vi "Test Create (From VI Reference).vi"(8 "error in (no error)":errorcluster) -> (0 "error out":errorcluster)   [LabVIEW 2020, in "TEST JKI State Machine API.lvlib"]
uses:
  TEST JKI State Machine API.lvlib
  <vilib>/addons/_JKI Toolkits/Caraya/classes/Assert/Assert.lvclass
  <vilib>/addons/_JKI Toolkits/Caraya/classes/Test/Test.lvclass
  source/JKI SM/JKI SM.lvclass
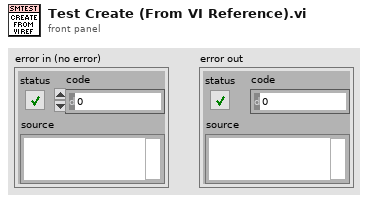
[diagram p1: front panel]
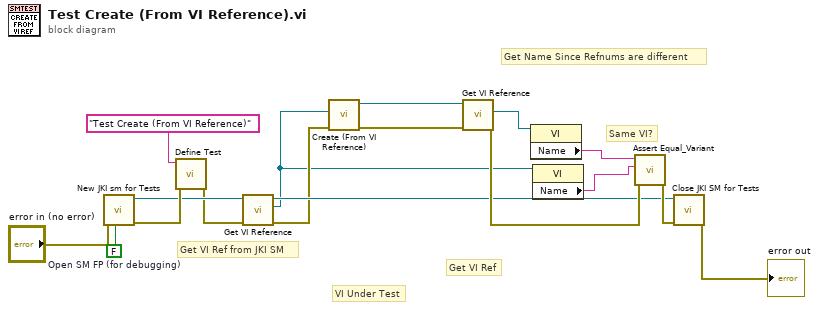
[diagram p0: block diagram]
diagram:
  w7 = FALSE  # Open SM FP (for debugging)
  # "Get Name Since Refnums are different"
  # "Get VI Ref"
  # "VI Under Test"
  # "Same VI?"
  # "Get VI Ref from JKI SM"
  n1 = call "New JKI sm for Tests.vi"("Open SM FP (for debugging)"=w7, "error in (no error)"="error in (no error)") -> ("error out"=w17:errorcluster, "JKI SM out"=w14:refnum<class "JKI SM.lvclass">)  [unwired: 8 in]
  n2 = call <vilib>:"Define Test.vi"("error in (no error)"=w17, "Label (VI Title)"="Test Create (From VI Reference)") -> ("error out"=w13:errorcluster)  [unwired: 8 in, 1 out]
  n3 = call "Get VI Reference.vi"("error in (no error)"=w13, "JKI SM in"=w14) -> ("error out"=w8:errorcluster, "VI"=w1:refnum<vi>, "JKI SM out"=w10:refnum<class "JKI SM.lvclass">)  [unwired: 7 in]
  n4 = call "Create (From VI Reference).vi"("error in (no error)"=w8, "VI"=w1) -> ("error out"=w12:errorcluster, "JKI SM out"=w9:refnum<class "JKI SM.lvclass">)  [unwired: 8 in]
  n5 = call "Get VI Reference.vi"("error in (no error)"=w12, "JKI SM in"=w9) -> ("error out"=w11:errorcluster, "VI"=w6:refnum<vi>)  [unwired: 7 in, 1 out]
  n6 = property class="VI"(reference=w6) -> ("Name"=w5:string)  [unwired: 1 in, 2 out]
  n7 = property class="VI"(reference=w1) -> ("Name"=w4:string)  [unwired: 1 in, 2 out]
  n8 = call <vilib>:"Assert Equal_Variant.vi"("error in (no error)"=w11, "Y"=w4, "X"=w5) -> ("error out"=w15:errorcluster)  [unwired: 8 in]
  n9 = call "Close JKI SM for Tests.vi"("error in (no error)"=w15, "JKI SM in"=w10) -> ("error out"=→"error out":errorcluster)  [unwired: 9 in]
